vi "openbci_start.vi"(8 "error in (no error)":errorcluster, 11 "OBCI dev in":T1={"COM port"="", "n_ch (8)"=enum."8 Channels", "delay_tx"=50}) -> (0 "error out":errorcluster, 3 "OBCI dev out":T1={"COM port"="", "n_ch (8)"=enum."8 Channels", "delay_tx"=50})   [LabVIEW 2013]
doc: "'b' Begin streaming data"
uses:
  Control Def/openbci_device.ctl
  Control Def/channel_count.ctl
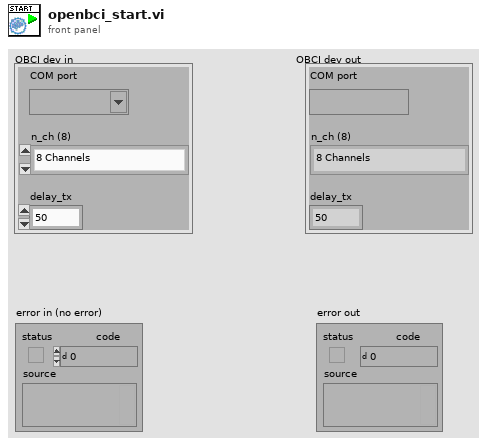
[diagram p1: front panel]
types:
  T1 = typedef "openbci_device.ctl" = cluster{"COM port":refnum<visa-resource-name>, "n_ch (8)":T2, "delay_tx":u32}
  T2 = typedef "channel_count.ctl" = enum16{"8 Channels", "16 Channels"}
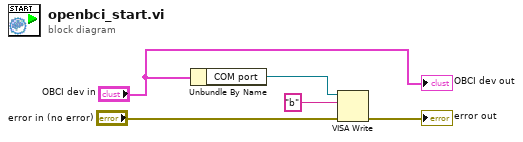
[diagram p0: block diagram]
diagram:
  n1 = Unbundle By Name("OBCI dev in") -> ("COM port"=w4:refnum<visa-resource-name>)
  n2 = VISA Write(VISA resource name=w4, write buffer="b", error in (no error)="error in (no error)") -> (error out=→"error out":errorcluster)  [unwired: 2 out]
  "OBCI dev out" <- "OBCI dev in"
